vi "GetAll Testbed.vi"() -> ()   [LabVIEW 2020, in "ORM_Examples.lvlib"]
uses:
  ORM_Examples.lvlib
  <vilib>/Viviota/shared/ORM_DBC_Sqlite.lvlibp/DBC.lvclass
  C:/Program Files/National Instruments/LabVIEW 2024/vi.lib/Viviota/shared/ORM.lvlibp/ORM/DbConnection/DbConnection.lvclass
  <vilib>/Viviota/shared/ORM.lvlibp/ORM/SqlMapper/SqlMapper.lvclass
  AlbumMap/AlbumMap.lvclass
  C:/Program Files/National Instruments/LabVIEW 2024/vi.lib/Viviota/shared/ORM.lvlibp/ORM/TypeMap/TypeMap.lvclass
  Album/Album.lvclass
  <vilib>/Viviota/shared/ORM_ADONet.lvlibp/ADOMapper/ADOMapper.lvclass
  C:/Program Files/National Instruments/LabVIEW 2024/vi.lib/Viviota/shared/ORM.lvlibp/ORM/SqlMapper/SqlMapper.lvclass
  Album/Album.lvclass/Album.ctl
  4d5a9e78-b4b3-4b9f-bd01-c943243a9c7d.vi
  Album/Read Primary Key.vi
  Album/Read Title.vi
  4d5a9e78-b4b3-4b9f-bd01-c943243a9c7d.vi/a9ccc3c9-891a-4d80-8d4f-837bdef88ccd.vi
  4d5a9e78-b4b3-4b9f-bd01-c943243a9c7d.vi/8216614f-f413-45b3-8111-14f8d0271ea5.vi
  4d5a9e78-b4b3-4b9f-bd01-c943243a9c7d.vi/fc6a5c23-d21f-4d2c-895e-66da96fa9491.vi
  4d5a9e78-b4b3-4b9f-bd01-c943243a9c7d.vi/fc6a5c23-d21f-4d2c-895e-66da96fa9491.vi/9d007ba8-e96f-4737-8d8a-6b46cf7f5c4a.vi
  4d5a9e78-b4b3-4b9f-bd01-c943243a9c7d.vi/fc6a5c23-d21f-4d2c-895e-66da96fa9491.vi/050765a8-e5d4-4415-b637-62775228e838.vi
  <vilib>/Viviota/shared/ORM.lvlibp/ORM/SqlMapper/Write DbConnection.vi
  <vilib>/Utility/error.llb/Error Cluster From Error Code.vi
  <vilib>/Viviota/shared/ORM.lvlibp/ORM/TypeMap/Read TypeMap.vi
  <vilib>/Viviota/shared/ORM.lvlibp/ORM/Query Result/Next.vi
  <vilib>/Viviota/shared/ORM.lvlibp/ORM/TypeMap/ToLabVIEW_Wrap.vi
  <vilib>/Viviota/shared/ORM.lvlibp/ORM/SqlMapper/End Transaction.vi
  <vilib>/Viviota/shared/ORM.lvlibp/ORM/TypeMap/TypeMap.lvclass
  <vilib>/Viviota/shared/ORM.lvlibp/ORM/Query Result/Query Result.lvclass
panel:
  out "Array":cluster{"Primary Key":i64, "Title":string}[](array[cluster])
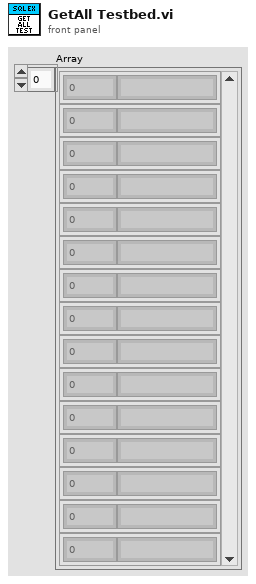
[diagram p1: front panel]
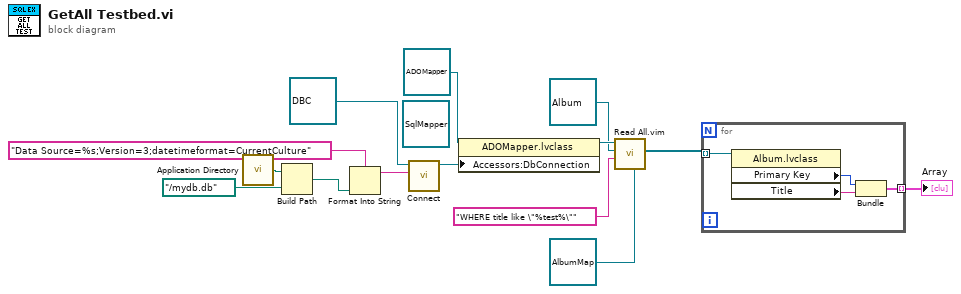
[diagram p0: block diagram]
diagram:
  (unwired) refnum<class "SqlMapper.lvclass"> refnum ("Dapper.lvlib:SqlMapper.lvclass")
  n1 = call <vilib>:"Application Directory.vi"() -> ("Application Directory"=w11:path)
  n2 = Build Path(base path=w11, name or relative path=path "../mydb.db" ("file out")) -> (appended path=w10:path)
  n3 = Format Into String(format string="Data Source=%s;Version=3;datetimeformat=CurrentCulture" ("connectionStringName"), w10) -> (resulting string=w9:string)  [unwired: 2 in, 1 out]
  n4 = call-dynamic "Connect.vi"("Connection String"=w9, "SqliteConnection in"=refnum<class "DBC.lvclass"> refnum) -> ("SqliteConnection out"=w8:refnum<class "DBC.lvclass">)  [unwired: 8 in, 1 out]
  n5 = property class="ADOMapper.lvclass"(reference=refnum<class "ADOMapper.lvclass"> refnum ("ADONet.lvlib:ADOMapper.lvclass"), "Accessors:DbConnection"=w8) -> (reference out=w7:refnum<class "ADOMapper.lvclass">)  [unwired: 1 in, 1 out]
  n6 = call "Read All.vim"("TypeMap in"=refnum<class "AlbumMap.lvclass"> refnum ("AlbumMap.lvclass"), "WHERE"="WHERE title like \"%test%\"", "Object"=refnum<class "Album.lvclass"> refnum ("Album.lvclass"), "SqlMapper in"=w7) -> ("Query Results"=w1:refnum<class "Album.lvclass">[])  [unwired: 5 in, 2 out]
  n7 = for {
    tunnel: w1 -> [w18] mode=indexing
    tunnel: [w15] -> w5 mode=indexing
    n8 = property class="Album.lvclass"(reference=w18) -> ("Primary Key"=w17:i64, "Title"=w16:string)  [unwired: 1 in, 2 out]
    n9 = Bundle("Primary Key"=w17, "Title"=w16) -> (w15:cluster{"Primary Key":i64, "Title":string})  [unwired: 1 in]
  }
  "Array" <- w5
